vi "AquireTape.vi"(8 "error in (no error)":errorcluster, 10 "Settings":T1={"max velocity"={"Value"=0.0, "Min"=0.0, "Max"=0.0, "StepSize"=0.0, "Tolerance"=0.0, "valueactual"=0.0}, "continious velocity"={"Value"=0.0, "Min"=0.0, "Max"=0.0, "StepSize"=0.0, "Tolerance"=0.0, "valueactual"=0.0}, "shake"=enum."off", "direction"=enum."left", "RedRatio"={"Value"=0.0, "Min"=0.0, "Max"=0.0, "StepSize"=0.0, "Tolerance"=0.0, "valueactual"=0.0}, "StepSize"={"Value"=0.0, "Min"=0.0, "Max"=0.0, "StepSize"=0.0, "Tolerance"=0.0, "valueactual"=0.0}, "position"={"Value"=0.0, "Min"=0.0, "Max"=0.0, "StepSize"=0.0, "Tolerance"=0.0, "valueactual"=0.0}, "velocity"={"Value"=0.0, "Min"=0.0, "Max"=0.0, "StepSize"=0.0, "Tolerance"=0.0, "valueactual"=0.0}, "Step"=enum."off", "Mode"=enum."on demand", "timeout"={"Value"=0.0, "Min"=0.0, "Max"=0.0, "StepSize"=0.0, "Tolerance"=0.0, "valueactual"=0.0}, "DelayStage"={"Value"=0.0, "Min"=0.0, "Max"=0.0, "StepSize"=0.0, "Tolerance"=0.0, "valueactual"=0.0}, "TapeMotor"=enum."off", "encoder Axis"=2, "oldpos"=0.0, "ResetEncoder"=enum."off"}, 11 "VISA Refnum in":refnum<visa-resource-name>) -> (0 "error out":errorcluster, 1 "RedRatio":dbl, 2 "Settings":T1={"max velocity"={"Value"=0.0, "Min"=0.0, "Max"=0.0, "StepSize"=0.0, "Tolerance"=0.0, "valueactual"=0.0}, "continious velocity"={"Value"=0.0, "Min"=0.0, "Max"=0.0, "StepSize"=0.0, "Tolerance"=0.0, "valueactual"=0.0}, "shake"=enum."off", "direction"=enum."left", "RedRatio"={"Value"=0.0, "Min"=0.0, "Max"=0.0, "StepSize"=0.0, "Tolerance"=0.0, "valueactual"=0.0}, "StepSize"={"Value"=0.0, "Min"=0.0, "Max"=0.0, "StepSize"=0.0, "Tolerance"=0.0, "valueactual"=0.0}, "position"={"Value"=0.0, "Min"=0.0, "Max"=0.0, "StepSize"=0.0, "Tolerance"=0.0, "valueactual"=0.0}, "velocity"={"Value"=0.0, "Min"=0.0, "Max"=0.0, "StepSize"=0.0, "Tolerance"=0.0, "valueactual"=0.0}, "Step"=enum."off", "Mode"=enum."on demand", "timeout"={"Value"=0.0, "Min"=0.0, "Max"=0.0, "StepSize"=0.0, "Tolerance"=0.0, "valueactual"=0.0}, "DelayStage"={"Value"=0.0, "Min"=0.0, "Max"=0.0, "StepSize"=0.0, "Tolerance"=0.0, "valueactual"=0.0}, "TapeMotor"=enum."off", "encoder Axis"=2, "oldpos"=0.0, "ResetEncoder"=enum."off"}, 3 "VISA Refnum out":refnum<visa-resource-name>, 4 "Position (units)":dbl, 6 "velocity":dbl)   [LabVIEW 2011]
uses:
  TapeDrive/settings_TypDef.ctl
  shared/numericVariable_TypeDef.ctl
  shared/OnOffTypeDef.ctl
  TapeDrive/Direction_TypDef.ctl
  TapeDrive/Mode_TypDEf.ctl
  shared/CompressAndUpdate(Poly)/CompressAndUpdate(Numeric).vi
  <instrlib>/Newport ESP301/Newport ESP301.lvlib
  TapeDrive/TapeDrive.lvclass
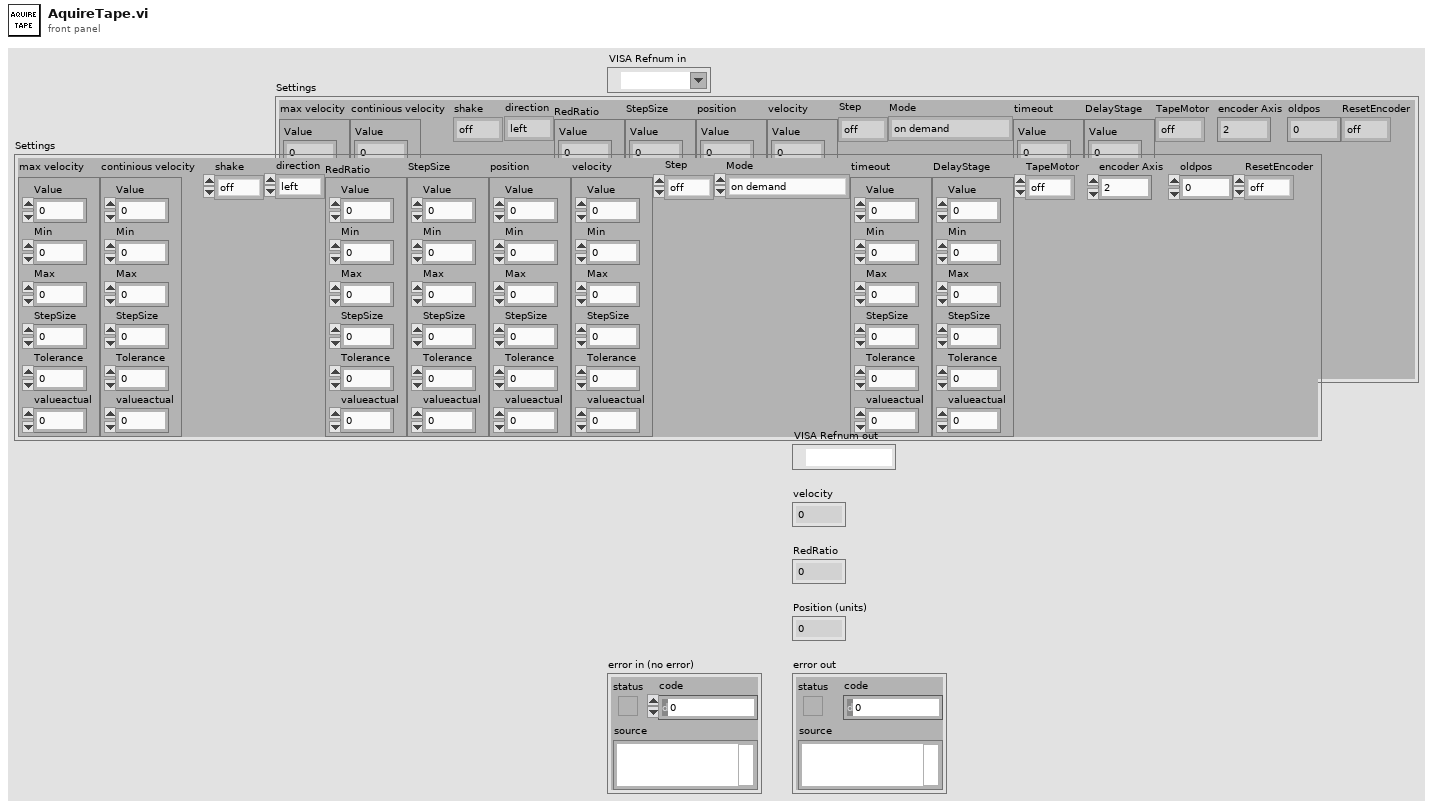
[diagram p1: front panel]
types:
  T1 = typedef "TapeDrive.lvclass/settings_TypDef.ctl" = cluster{"max velocity":T2, "continious velocity":T2, "shake":T3, "direction":T4, "RedRatio":T2, "StepSize":T2, "position":T2, "velocity":T2, "Step":T3, "Mode":T5, "timeout":T2, "DelayStage":T2, "TapeMotor":T3, "encoder Axis":i32, "oldpos":dbl, "ResetEncoder":T3}
  T2 = typedef "numericVariable_TypeDef.ctl" = cluster{"Value":dbl, "Min":dbl, "Max":dbl, "StepSize":dbl, "Tolerance":dbl, "valueactual":dbl}
  T3 = typedef "OnOffTypeDef.ctl" = enum16{"off", "on"}
  T4 = typedef "Direction_TypDef.ctl" = enum16{"left", "right"}
  T5 = typedef "Mode_TypDEf.ctl" = enum16{"on demand", "continuous", "scan"}
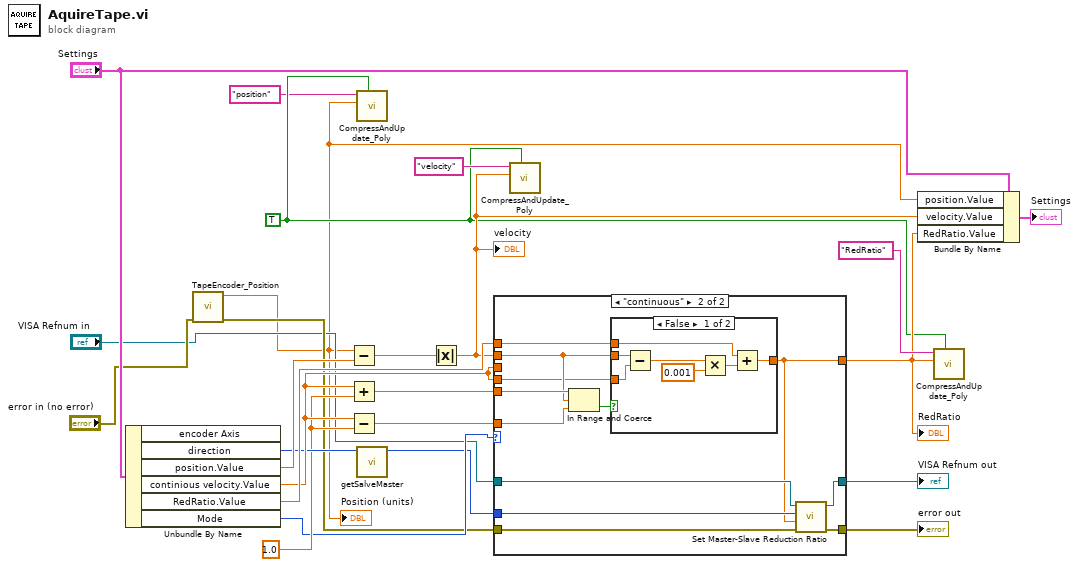
[diagram p0: block diagram]
diagram:
  w8 = TRUE ("force CVT update (false)")
  w16 = 1.0 ("y")
  n1 = Unbundle By Name("Settings") -> ("direction"=w19:T4, "position.Value"=w20:dbl, "continious velocity.Value"=w22:dbl, "RedRatio.Value"=w24:dbl, "Mode"=w6:T5)  [unwired: 1 out]
  n2 = call "TapeEncoder_Position.vi"("error in (no error)"="error in (no error)") -> ("error IO"=w3:errorcluster, "position"=w1:dbl)  [unwired: 9 in]
  "Position (units)" <- w1
  n3 = Subtract(x=w1, y=w20) -> (x-y=w13:dbl)
  n4 = Add(x=w22, y=w16) -> (x+y=w17:dbl)
  n5 = Subtract(x=w22, y=w16) -> (x-y=w18:dbl)
  n6 = call-poly "CompressAndUpdate_Poly.vi"("force CVT update (false)"=w8, "Numeric"=w1, "command or variable name"="position") -> ()  [unwired: 8 in, 1 out]
  n7 = call "getSalveMaster.vi"("direction"=w19) -> ("Slave"=w5:i32)  [unwired: 9 in, 1 out]
  n8 = Absolute Value(x=w13) -> (abs(x)=w11:dbl)
  "velocity" <- w11
  n9 = case shown="\"continuous\"" w6 {
    tunnel: "VISA Refnum in" -> [w27 w39]
    tunnel: [w27 w38] -> w14
    tunnel: w3 -> [w26 w37]
    tunnel: [w26 w36] -> w15
    tunnel: w5 -> [_ w35]
    tunnel: w22 -> [_ _]
    tunnel: w11 -> [_ w31]
    tunnel: w17 -> [_ w34]
    tunnel: w18 -> [_ w33]
    tunnel: w22 -> [_ w30]
    tunnel: w24 -> [w25 w29]
    tunnel: [w25 w28] -> w9
    frame "on demand", Default {
    }
    frame "continuous" {
      n10 = In Range and Coerce(upper limit=w34, x=w31, lower limit=w33) -> (In Range?=w32:bool)  [unwired: 1 out]
      n11 = case shown="False" w32 {
        tunnel: w31 -> [w46 _]
        tunnel: w30 -> [w45 _]
        tunnel: [w41 w47] -> w28
        tunnel: w29 -> [w40 w47]
        frame False {
          n12 = Subtract(x=w46, y=w45) -> (x-y=w44:dbl)
          n13 = Multiply(x=w44, y=0.001) -> (x*y=w42:dbl)
          n14 = Add(x=w40, y=w42) -> (x+y=w41:dbl)
        }
        frame True {
        }
      }
      n15 = call <instrlib>:"Set Master-Slave Reduction Ratio.vi"("error in (no error)"=w37, "Reduction Ratio (0)"=w28, "Axis (1)"=w35, "VISA resource name"=w39) -> ("error out"=w36:errorcluster, "VISA resource name out"=w38:refnum<visa-resource-name>)  [unwired: 2 in]
    }
  }
  "RedRatio" <- w9
  "error out" <- w15
  "VISA Refnum out" <- w14
  n16 = call-poly "CompressAndUpdate_Poly.vi"("force CVT update (false)"=w8, "Numeric"=w11, "command or variable name"="velocity") -> ()  [unwired: 8 in, 1 out]
  n17 = Bundle By Name(cluster="Settings", "position.Value"=w1, "velocity.Value"=w11, "RedRatio.Value"=w9) -> (→"Settings":T1)
  n18 = call-poly "CompressAndUpdate_Poly.vi"("force CVT update (false)"=w8, "Numeric"=w9, "command or variable name"="RedRatio") -> ()  [unwired: 8 in, 1 out]
